vi "fpga_I32xU32 MAC (MSBs).vi"(1 "sum[I32]":i32, 2 "y[U32]":u32, 3 "x[I32]":i32) -> (0 "x*y+sum[I32 MSB]":i32)   [LabVIEW 2011, in "NI_EP_Resample_FPGA.lvlib"]
uses:
  <vilib>/rvi/Arithmetic/AddSubMult/XNode/nirviSatArithmetic.xnode
  <vilib>/addons/Electrical Power/PQ/Resampling/NI_EP_Resample_FPGA.lvlib
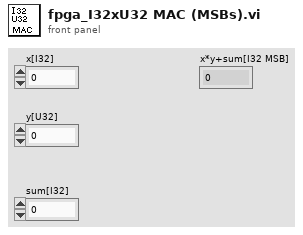
[diagram p1: front panel]
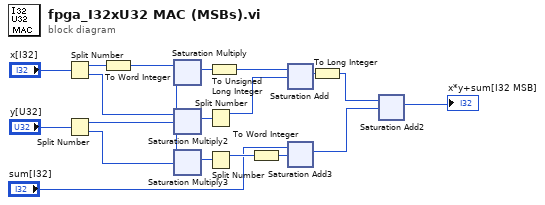
[diagram p0: block diagram]
diagram:
  n1 = Split Number(x="x[I32]") -> (hi(x)=w11:u16, lo(x)=w16:u16)
  n2 = Split Number(x="y[U32]") -> (hi(x)=w14:u16, lo(x)=w13:u16)
  n3 = To Word Integer(number=w11) -> (16bit integer=w8:i16)
  n4 = xnode ("Saturation Multiply")("x"=w8, "y"=w14) -> ("x*y"=w7:i32)
  n5 = xnode ("Saturation Multiply2")("x"=w16, "y"=w14) -> ("x*y"=w17:u32)
  n6 = xnode ("Saturation Multiply3")("x"=w8, "y"=w13) -> ("x*y"=w12:i32)
  n7 = Split Number(x=w17) -> (hi(x)=w18:u16)  [unwired: 1 out]
  n8 = Split Number(x=w12) -> (hi(x)=w9:u16)  [unwired: 1 out]
  n9 = To Unsigned Long Integer(number=w7) -> (unsigned 32bit integer=w6:u32)
  n10 = To Word Integer(number=w9) -> (16bit integer=w2:i16)
  n11 = xnode ("Saturation Add")("x"=w6, "y"=w18) -> ("x+y"=w10:u32)
  n12 = xnode ("Saturation Add3")("x"="sum[I32]", "y"=w2) -> ("x+y"=w1:i32)
  n13 = To Long Integer(number=w10) -> (32bit integer=w5:i32)
  n14 = xnode ("Saturation Add2")("x"=w5, "y"=w1) -> ("x+y"=→"x*y+sum[I32 MSB]":i32)
